vi "createEvent.vi"(8 "error in (no error)":errorcluster, 11 "Handler.UserEvent.Console in":refnum<class "Handler.UserEvent.Console.lvclass">) -> (0 "error out":errorcluster, 3 "Handler.UserEvent.Console out":refnum<class "Handler.UserEvent.Console.lvclass">)   [LabVIEW 2017, in "Error Log.lvlib" / "Handler.UserEvent.Console.lvclass"]
uses:
  Handler.UserEvent.Console.lvclass
  Handler.UserEvent.Console.lvclass/Handler.UserEvent.Console.ctl
  Handler.UserEvent/Handler.UserEvent.lvclass
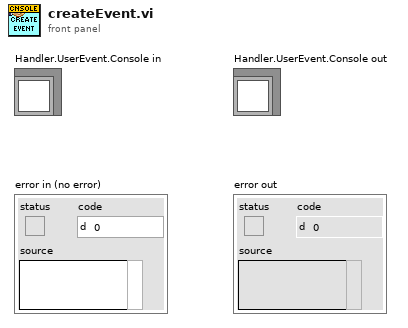
[diagram p1: front panel]
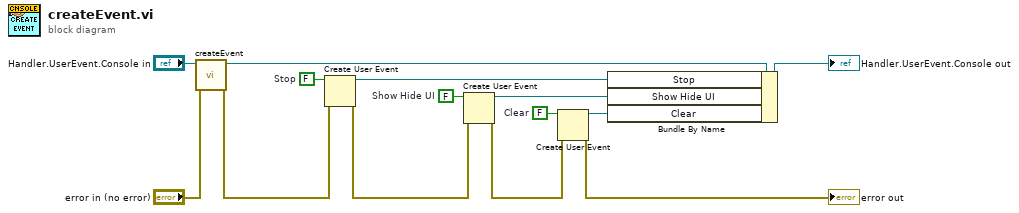
[diagram p0: block diagram]
diagram:
  w4 = FALSE  # Clear
  w10 = FALSE  # Stop
  w11 = FALSE  # Show Hide UI
  n1 = call-parent "createEvent.vi"("error in (no error)"="error in (no error)", "Handler.UserEvent in"="Handler.UserEvent.Console in") -> ("error out"=w5:errorcluster, "Handler.UserEvent out"=w14:refnum<class "Handler.UserEvent.Console.lvclass">)  [unwired: 8 in]
  n2 = Create User Event(user event datatype=w10, error in=w5) -> (user event=w8:refnum<user-event>, error out=w6:errorcluster)
  n3 = Create User Event(user event datatype=w11, error in=w6) -> (user event=w7:refnum<user-event>, error out=w2:errorcluster)
  n4 = Create User Event(user event datatype=w4, error in=w2) -> (user event=w3:refnum<user-event>, error out=→"error out":errorcluster)
  n5 = Bundle By Name(cluster=w14, "Stop"=w8, "Show Hide UI"=w7, "Clear"=w3) -> (→"Handler.UserEvent.Console out":refnum<class "Handler.UserEvent.Console.lvclass">)
